vi "Untitled 3.vi"() -> ()   [LabVIEW 2018]
panel:
  in  "Numeric 2":dbl
  in  "stop":bool
  out "Numeric":dbl format="%#_3g"
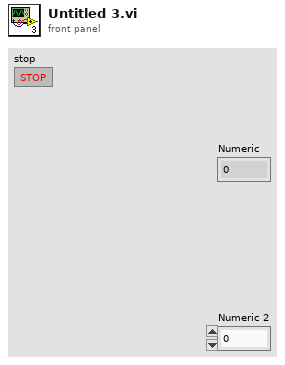
[diagram p1: front panel]
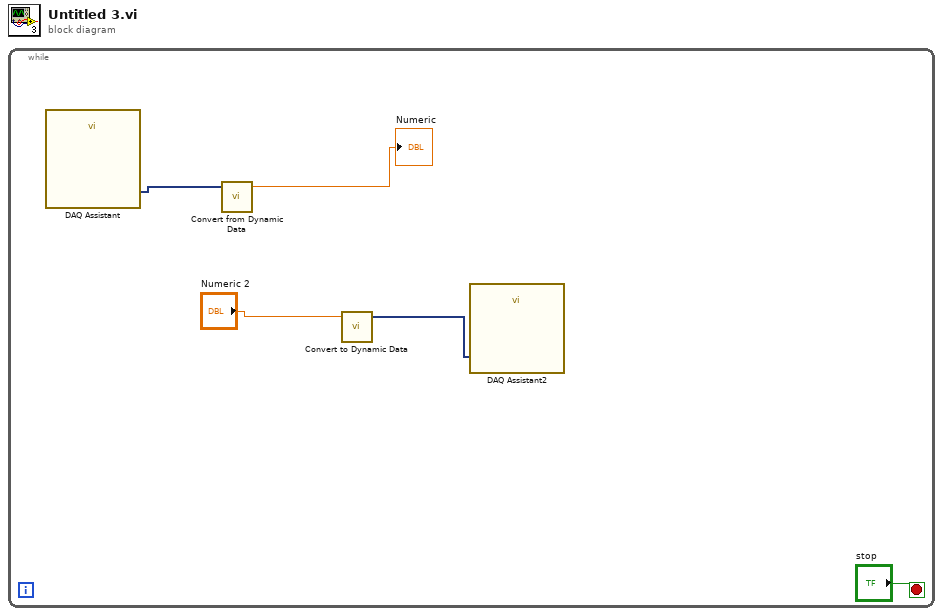
[diagram p0: block diagram]
diagram:
  n1 = while {
    stop <- "stop" stop-if-true
    n2 = call "DAQ Assistant"() -> ("data"=w5:dynamicdata)  [unwired: 17 in, 2 out]
    n3 = call "Convert from Dynamic Data"("Dynamic Data Type"=w5) -> ("Scalar"=→"Numeric":dbl)  [unwired: 3 in]
    n4 = call "Convert to Dynamic Data"("Double"="Numeric 2") -> ("Dynamic Data Type"=w1:dynamicdata)  [unwired: 3 in]
    n5 = call "DAQ Assistant2"("data"=w1) -> ()  [unwired: 17 in, 2 out]
  }
